vi "siglent_config.vi"(8 "error in (no error)":errorcluster, 10 "Kalibracni bod":T1, 11 "VISA Refnum in":refnum<visa-resource-name>) -> (0 "error out":errorcluster, 3 "VISA Refnum out":refnum<visa-resource-name>)   [LabVIEW 2022 SP3]
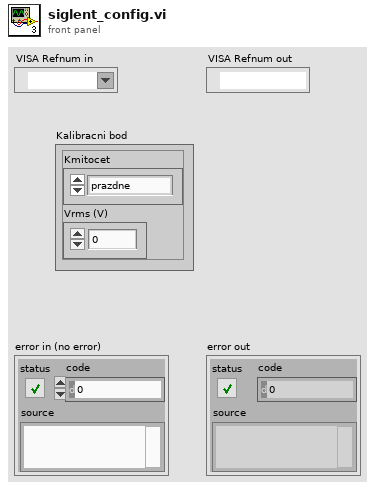
[diagram p1: front panel]
types:
  T1 = cluster{"Kmitocet":enum16{"prazdne", "50 Hz", "1 kHz", "5 kHz", "10 kHz", "20 kHz", "50 kHz", "100 kHz"}, "Vrms (V)":dbl}
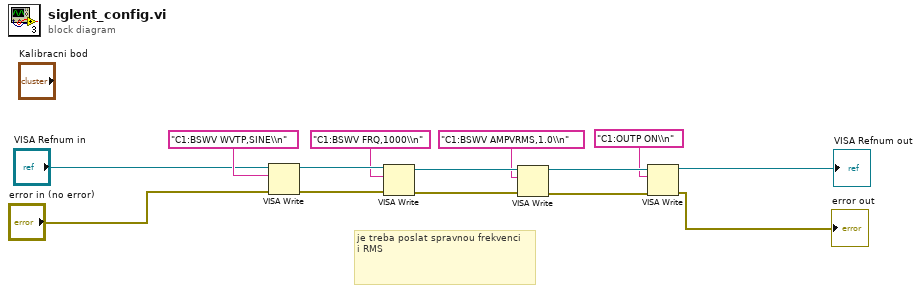
[diagram p0: block diagram]
diagram:
  # "je treba poslat spravnou frekvenci\ni RMS"
  n1 = VISA Write(VISA resource name="VISA Refnum in", write buffer="C1:BSWV WVTP,SINE\\n", error in (no error)="error in (no error)") -> (VISA resource name out=w5:refnum<visa-resource-name>, error out=w6:errorcluster)  [unwired: 1 out]
  n2 = VISA Write(VISA resource name=w5, write buffer="C1:BSWV FRQ,1000\\n", error in (no error)=w6) -> (VISA resource name out=w8:refnum<visa-resource-name>, error out=w9:errorcluster)  [unwired: 1 out]
  n3 = VISA Write(VISA resource name=w8, write buffer="C1:BSWV AMPVRMS,1.0\\n", error in (no error)=w9) -> (VISA resource name out=w12:refnum<visa-resource-name>, error out=w11:errorcluster)  [unwired: 1 out]
  n4 = VISA Write(VISA resource name=w12, write buffer="C1:OUTP ON\\n", error in (no error)=w11) -> (VISA resource name out=→"VISA Refnum out":refnum<visa-resource-name>, error out=→"error out":errorcluster)  [unwired: 1 out]
